vi "Turn on_off heating 4 vessel (SILAR).vi"(0 "Arduino Resource In 1":T1={"VISA resource"="", "Board Type"=enum."Uno", "Connection Type"=enum."USB / Serial", "Bytes Per Packet (15)"=15}, 7 "Error In 1":errorcluster, 13 "t1 - время во включенном состоянии":dbl[](array[numeric])) -> (20 "Arduino Resource Out 1":T1={"VISA resource"="", "Board Type"=enum."Uno", "Connection Type"=enum."USB / Serial", "Bytes Per Packet (15)"=15}, 21 "error out 1":errorcluster, 22 "Arduino Resource Out 2":T1={"VISA resource"="", "Board Type"=enum."Uno", "Connection Type"=enum."USB / Serial", "Bytes Per Packet (15)"=15}, 23 "error out 2":errorcluster, 24 "Arduino Resource Out 3":T1={"VISA resource"="", "Board Type"=enum."Uno", "Connection Type"=enum."USB / Serial", "Bytes Per Packet (15)"=15}, 25 "error out 3":errorcluster, 26 "Arduino Resource Out 4":T1={"VISA resource"="", "Board Type"=enum."Uno", "Connection Type"=enum."USB / Serial", "Bytes Per Packet (15)"=15}, 27 "error out 4":errorcluster)   [LabVIEW 2016]
uses:
  <vilib>/LabVIEW Interface for Arduino/Type Defs/Arduino Resource.ctl
  <vilib>/LabVIEW Interface for Arduino/Type Defs/Board Type.ctl
  <vilib>/LabVIEW Interface for Arduino/LabVIEW Interface for Arduino.lvlib
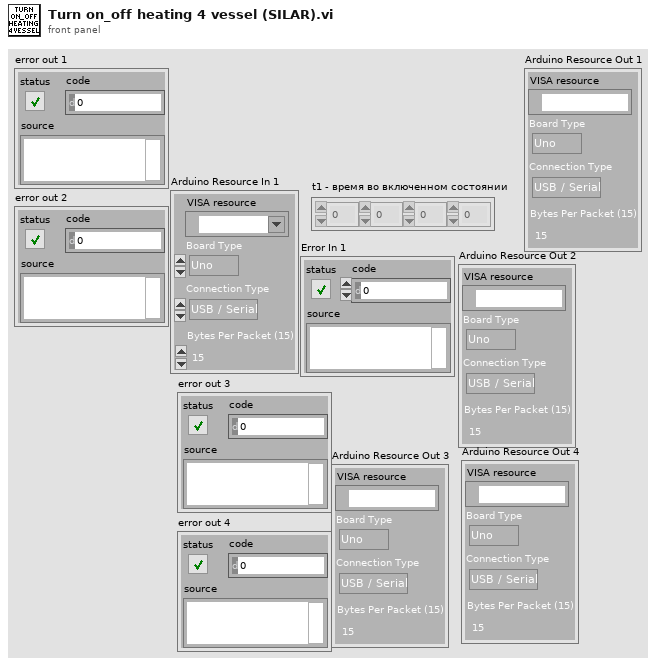
[diagram p1: front panel]
types:
  T1 = typedef "LabVIEW Interface for Arduino.lvlib/Arduino Resource.ctl" = cluster{"VISA resource":refnum<visa-resource-name>, "Board Type":T2, "Connection Type":enum8{"USB / Serial"}, "Bytes Per Packet (15)":u8}
  T2 = typedef "LabVIEW Interface for Arduino.lvlib/Board Type.ctl" = enum16{"Uno", "Dimuelanove w/Atmega 328", "Mega 2560"}
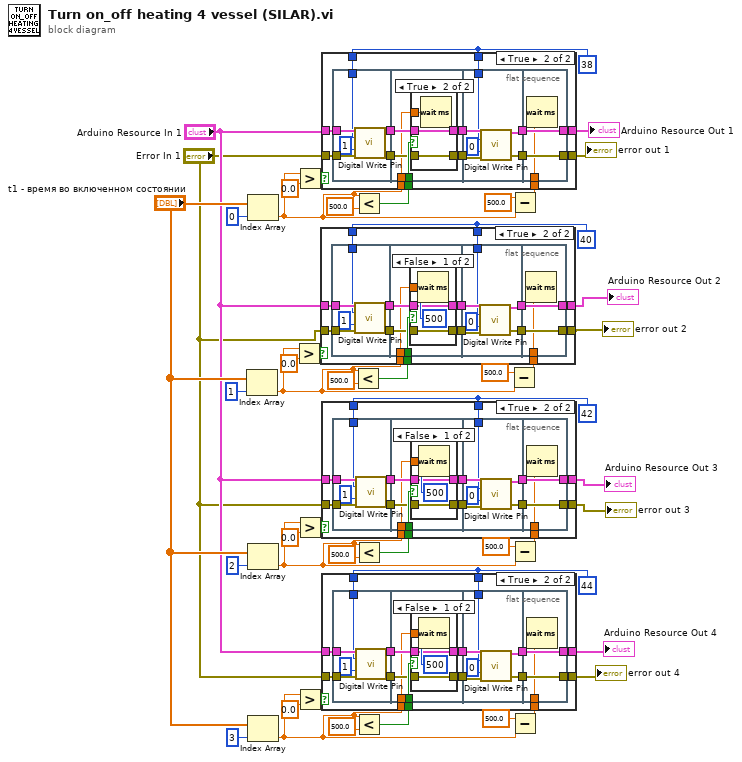
[diagram p0: block diagram]
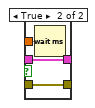
[diagram p3: hidden frame]
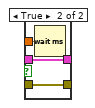
[diagram p5: hidden frame]
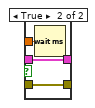
[diagram p7: hidden frame]
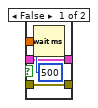
[diagram p9: hidden frame]
diagram:
  w14 = u8 44 ("Digital I/O Pin (0) 4")
  w23 = u8 42 ("Digital I/O Pin (0) 4")
  w32 = u8 40 ("Digital I/O Pin (0) 4")
  w41 = u8 38 ("Digital I/O Pin (0) 4")
  n1 = Index Array(array="t1 - время во включенном состоянии", index=1) -> (element=w30:dbl)
  n2 = Index Array(array="t1 - время во включенном состоянии", index=0) -> (element=w39:dbl)
  n3 = Index Array(array="t1 - время во включенном состоянии", index=2) -> (element=w21:dbl)
  n4 = Index Array(array="t1 - время во включенном состоянии", index=3) -> (element=w12:dbl)
  n5 = Greater?(x=w30, y=0.0) -> (0:w35:bool)
  n6 = Greater?(x=w39, y=0.0) -> (0:w44:bool)
  n7 = Greater?(x=w21, y=0.0) -> (0:w26:bool)
  n8 = Greater?(x=w12, y=0.0) -> (0:w17:bool)
  n9 = Less?(x=w30, y=500.0) -> (x < y?=w34:bool)
  n10 = Less?(x=w39, y=500.0) -> (x < y?=w43:bool)
  n11 = Less?(x=w21, y=500.0) -> (x < y?=w25:bool)
  n12 = Less?(x=w12, y=500.0) -> (x < y?=w16:bool)
  n13 = Subtract(x=500.0, y=w30) -> (x-y=w33:dbl)
  n14 = case shown="True" w35 {
    tunnel: "Error In 1" -> [w48 w62]
    tunnel: "Arduino Resource In 1" -> [w49 w61]
    tunnel: [w49 w60] -> w7
    tunnel: [w48 w59] -> w1
    tunnel: w30 -> [_ w52]
    tunnel: w34 -> [_ w55]
    tunnel: w33 -> [_ w53]
    tunnel: w32 -> [_ w51]
    tunnel: w32 -> [_ w50]
    frame False {
    }
    frame True {
      n15 = flat-sequence {
        tunnel: w62 -> [w70]
        tunnel: w61 -> [w69]
        tunnel: [w68] -> w64
        tunnel: [w67] -> w63
        tunnel: w51 -> [w65]
        tunnel: w64 -> [w75]
        tunnel: w63 -> [w73]
        tunnel: [w74] -> w58
        tunnel: w55 -> [w76]
        tunnel: [w72] -> w54
        tunnel: w52 -> [w71]
        tunnel: w58 -> [w87]
        tunnel: [w86] -> w57
        tunnel: [w85] -> w56
        tunnel: w54 -> [w84]
        tunnel: w50 -> [w83]
        tunnel: [w90] -> w59
        tunnel: [w91] -> w60
        tunnel: w57 -> [w91]
        tunnel: w56 -> [w90]
        tunnel: w53 -> [w89]
        frame #0 {
          n16 = call <vilib>:"Digital Write Pin.vi"("Arduino Resource"=w69, "Digital I/O Pin (0)"=w65, "Value (0)"=u8 1, "error in"=w70) -> ("Arduino Resource"=w68:T1, "error out"=w67:errorcluster)  [unwired: 10 in]
        }
        frame #1 {
          n17 = case shown="False" w76 {
            tunnel: w71 -> [_ w82]
            tunnel: w75 -> [w78 w81]
            tunnel: [w78 w81] -> w74
            tunnel: w73 -> [w77 w80]
            tunnel: [w77 w80] -> w72
            frame False {
              n18 = Wait (ms)(milliseconds to wait=u32 500) -> ()  [unwired: 1 out]
            }
            frame True {
              n19 = Wait (ms)(milliseconds to wait=w82) -> ()  [unwired: 1 out]
            }
          }
        }
        frame #2 {
          n20 = call <vilib>:"Digital Write Pin.vi"("Arduino Resource"=w87, "Digital I/O Pin (0)"=w83, "Value (0)"=u8 0, "error in"=w84) -> ("Arduino Resource"=w86:T1, "error out"=w85:errorcluster)  [unwired: 10 in]
        }
        frame #3 {
          n21 = Wait (ms)(milliseconds to wait=w89) -> ()  [unwired: 1 out]
        }
      }
    }
  }
  "Arduino Resource Out 2" <- w7
  "error out 2" <- w1
  n22 = Subtract(x=500.0, y=w39) -> (x-y=w42:dbl)
  n23 = case shown="True" w44 {
    tunnel: "Error In 1" -> [w92 w106]
    tunnel: "Arduino Resource In 1" -> [w93 w105]
    tunnel: [w93 w104] -> w8
    tunnel: [w92 w103] -> w4
    tunnel: w39 -> [_ w96]
    tunnel: w43 -> [_ w99]
    tunnel: w42 -> [_ w97]
    tunnel: w41 -> [_ w95]
    tunnel: w41 -> [_ w94]
    frame False {
    }
    frame True {
      n24 = flat-sequence {
        tunnel: w106 -> [w114]
        tunnel: w105 -> [w113]
        tunnel: [w112] -> w108
        tunnel: [w111] -> w107
        tunnel: w95 -> [w109]
        tunnel: w108 -> [w119]
        tunnel: w107 -> [w117]
        tunnel: [w118] -> w102
        tunnel: w99 -> [w120]
        tunnel: [w116] -> w98
        tunnel: w96 -> [w115]
        tunnel: w102 -> [w131]
        tunnel: [w130] -> w101
        tunnel: [w129] -> w100
        tunnel: w98 -> [w128]
        tunnel: w94 -> [w127]
        tunnel: [w134] -> w103
        tunnel: [w135] -> w104
        tunnel: w101 -> [w135]
        tunnel: w100 -> [w134]
        tunnel: w97 -> [w133]
        frame #0 {
          n25 = call <vilib>:"Digital Write Pin.vi"("Arduino Resource"=w113, "Digital I/O Pin (0)"=w109, "Value (0)"=u8 1, "error in"=w114) -> ("Arduino Resource"=w112:T1, "error out"=w111:errorcluster)  [unwired: 10 in]
        }
        frame #1 {
          n26 = case shown="True" w120 {
            tunnel: w115 -> [_ w126]
            tunnel: w119 -> [w122 w125]
            tunnel: [w122 w125] -> w118
            tunnel: w117 -> [w121 w124]
            tunnel: [w121 w124] -> w116
            frame False {
              n27 = Wait (ms)(milliseconds to wait=u32 500) -> ()  [unwired: 1 out]
            }
            frame True {
              n28 = Wait (ms)(milliseconds to wait=w126) -> ()  [unwired: 1 out]
            }
          }
        }
        frame #2 {
          n29 = call <vilib>:"Digital Write Pin.vi"("Arduino Resource"=w131, "Digital I/O Pin (0)"=w127, "Value (0)"=u8 0, "error in"=w128) -> ("Arduino Resource"=w130:T1, "error out"=w129:errorcluster)  [unwired: 10 in]
        }
        frame #3 {
          n30 = Wait (ms)(milliseconds to wait=w133) -> ()  [unwired: 1 out]
        }
      }
    }
  }
  "Arduino Resource Out 1" <- w8
  "error out 1" <- w4
  n31 = Subtract(x=500.0, y=w21) -> (x-y=w24:dbl)
  n32 = case shown="True" w26 {
    tunnel: "Error In 1" -> [w136 w150]
    tunnel: "Arduino Resource In 1" -> [w137 w149]
    tunnel: [w137 w148] -> w6
    tunnel: [w136 w147] -> w2
    tunnel: w21 -> [_ w140]
    tunnel: w25 -> [_ w143]
    tunnel: w24 -> [_ w141]
    tunnel: w23 -> [_ w139]
    tunnel: w23 -> [_ w138]
    frame False {
    }
    frame True {
      n33 = flat-sequence {
        tunnel: w150 -> [w158]
        tunnel: w149 -> [w157]
        tunnel: [w156] -> w152
        tunnel: [w155] -> w151
        tunnel: w139 -> [w153]
        tunnel: w152 -> [w163]
        tunnel: w151 -> [w161]
        tunnel: [w162] -> w146
        tunnel: w143 -> [w164]
        tunnel: [w160] -> w142
        tunnel: w140 -> [w159]
        tunnel: w146 -> [w175]
        tunnel: [w174] -> w145
        tunnel: [w173] -> w144
        tunnel: w142 -> [w172]
        tunnel: w138 -> [w171]
        tunnel: [w178] -> w147
        tunnel: [w179] -> w148
        tunnel: w145 -> [w179]
        tunnel: w144 -> [w178]
        tunnel: w141 -> [w177]
        frame #0 {
          n34 = call <vilib>:"Digital Write Pin.vi"("Arduino Resource"=w157, "Digital I/O Pin (0)"=w153, "Value (0)"=u8 1, "error in"=w158) -> ("Arduino Resource"=w156:T1, "error out"=w155:errorcluster)  [unwired: 10 in]
        }
        frame #1 {
          n35 = case shown="False" w164 {
            tunnel: w159 -> [_ w170]
            tunnel: w163 -> [w166 w169]
            tunnel: [w166 w169] -> w162
            tunnel: w161 -> [w165 w168]
            tunnel: [w165 w168] -> w160
            frame False {
              n36 = Wait (ms)(milliseconds to wait=u32 500) -> ()  [unwired: 1 out]
            }
            frame True {
              n37 = Wait (ms)(milliseconds to wait=w170) -> ()  [unwired: 1 out]
            }
          }
        }
        frame #2 {
          n38 = call <vilib>:"Digital Write Pin.vi"("Arduino Resource"=w175, "Digital I/O Pin (0)"=w171, "Value (0)"=u8 0, "error in"=w172) -> ("Arduino Resource"=w174:T1, "error out"=w173:errorcluster)  [unwired: 10 in]
        }
        frame #3 {
          n39 = Wait (ms)(milliseconds to wait=w177) -> ()  [unwired: 1 out]
        }
      }
    }
  }
  "Arduino Resource Out 3" <- w6
  "error out 3" <- w2
  n40 = Subtract(x=500.0, y=w12) -> (x-y=w15:dbl)
  n41 = case shown="True" w17 {
    tunnel: "Error In 1" -> [w180 w194]
    tunnel: "Arduino Resource In 1" -> [w181 w193]
    tunnel: [w181 w192] -> w5
    tunnel: [w180 w191] -> w3
    tunnel: w12 -> [_ w184]
    tunnel: w16 -> [_ w187]
    tunnel: w15 -> [_ w185]
    tunnel: w14 -> [_ w183]
    tunnel: w14 -> [_ w182]
    frame False {
    }
    frame True {
      n42 = flat-sequence {
        tunnel: w194 -> [w202]
        tunnel: w193 -> [w201]
        tunnel: [w200] -> w196
        tunnel: [w199] -> w195
        tunnel: w183 -> [w197]
        tunnel: w196 -> [w207]
        tunnel: w195 -> [w205]
        tunnel: [w206] -> w190
        tunnel: w187 -> [w208]
        tunnel: [w204] -> w186
        tunnel: w184 -> [w203]
        tunnel: w190 -> [w219]
        tunnel: [w218] -> w189
        tunnel: [w217] -> w188
        tunnel: w186 -> [w216]
        tunnel: w182 -> [w215]
        tunnel: [w222] -> w191
        tunnel: [w223] -> w192
        tunnel: w189 -> [w223]
        tunnel: w188 -> [w222]
        tunnel: w185 -> [w221]
        frame #0 {
          n43 = call <vilib>:"Digital Write Pin.vi"("Arduino Resource"=w201, "Digital I/O Pin (0)"=w197, "Value (0)"=u8 1, "error in"=w202) -> ("Arduino Resource"=w200:T1, "error out"=w199:errorcluster)  [unwired: 10 in]
        }
        frame #1 {
          n44 = case shown="False" w208 {
            tunnel: w203 -> [_ w214]
            tunnel: w207 -> [w210 w213]
            tunnel: [w210 w213] -> w206
            tunnel: w205 -> [w209 w212]
            tunnel: [w209 w212] -> w204
            frame False {
              n45 = Wait (ms)(milliseconds to wait=u32 500) -> ()  [unwired: 1 out]
            }
            frame True {
              n46 = Wait (ms)(milliseconds to wait=w214) -> ()  [unwired: 1 out]
            }
          }
        }
        frame #2 {
          n47 = call <vilib>:"Digital Write Pin.vi"("Arduino Resource"=w219, "Digital I/O Pin (0)"=w215, "Value (0)"=u8 0, "error in"=w216) -> ("Arduino Resource"=w218:T1, "error out"=w217:errorcluster)  [unwired: 10 in]
        }
        frame #3 {
          n48 = Wait (ms)(milliseconds to wait=w221) -> ()  [unwired: 1 out]
        }
      }
    }
  }
  "Arduino Resource Out 4" <- w5
  "error out 4" <- w3
